vi "Configure Output Range Core.vi"(6 "range (0.0)":dbl format="%^.2e", 8 "error in (no error)":errorcluster, 9 "range type (Voltage)":i32(ring)=1 items=["Voltage"=1, "Current"=0], 10 "channel name (\"CHANNEL1\")":string="CHANNEL1", 11 "CS++DCPwr in":refnum<class "CS++DCPwr.lvclass">) -> (0 "error out":errorcluster, 3 "CS++DCPwr out":refnum<class "CS++DCPwr.lvclass">)   [LabVIEW 2016, in "CS++DCPwr.lvlib" / "CS++DCPwr.lvclass"]
doc: "Configures the power supply's output range on a channel. You specify whether you want to configure the voltage or current range, and the value to which to set the range.\n\nNotes:\n\n1) Setting a voltage range can invalidate a previously configured current range.\n\n2) Setting a current range can invalidate a previously configured voltage range."
uses:
  CS++DCPwr.lvclass
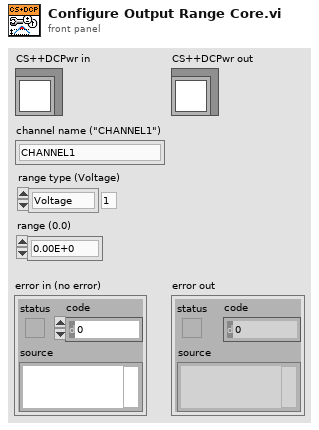
[diagram p1: front panel]
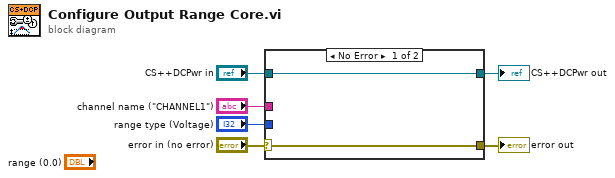
[diagram p0: block diagram]
diagram:
  n1 = case shown="No Error" "error in (no error)" {
    selector: "error in (no error)" -> [w7 w10]
    tunnel: [w7 w10] -> w5
    tunnel: [w8 w9] -> w3
    tunnel: "CS++DCPwr in" -> [w8 w9]
    tunnel: "channel name (\"CHANNEL1\")" -> [_ _]
    tunnel: "range type (Voltage)" -> [_ _]
    frame No Error {
    }
    frame Error {
    }
  }
  "error out" <- w5
  "CS++DCPwr out" <- w3
